vi "get day folder.vi"() -> (0 "error out":errorcluster, 3 "day folder":string[](array[string]))   [LabVIEW 2014]
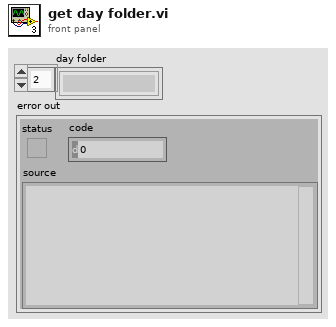
[diagram p1: front panel]
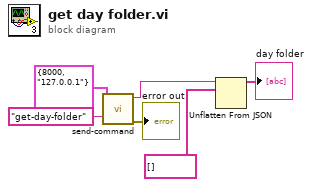
[diagram p0: block diagram]
diagram:
  n1 = call "send-command.vi"("command"="get-day-folder", "target"=cluster{"port":i32, "host":string} {"port"=8000, "host"="127.0.0.1"}) -> ("error out"=→"error out":errorcluster, "output"=w4:string)  [unwired: 8 in]
  n2 = Unflatten From JSON(JSON string=w4, type and defaults=string[] []) -> (value=→"day folder":string[])  [unwired: 5 in, 1 out]
